vi "air flow calibrator (source setpoint).vi"(4 "State":i16, 5 "Time":dbl format="%.2f", 6 "Sensor Values":dbl[](array[numeric])=[120000.0, 10000.0], 7 "Set Points":dbl[](array[numeric])=[1.0, 22.0, 5e-05]) -> (0 "required data":T1={"Set Point names"=["accumulator volume (L)", "air temperature (C)", "calibration state number", "Source pressure (Pa)"], "required number of setpoints"=4, "required number of sensors"=1, "Sensor names"=["Accumulator pressure (Pa)"]}, 3 "output value":dbl)   [LabVIEW 2019]
uses:
  <vilib>/Analysis/NI_AALPro.lvlib
panel:
  # "Enter the correct information for this control code in the required data structure below. Then make the current value default by right clicking on the border of the data structure."
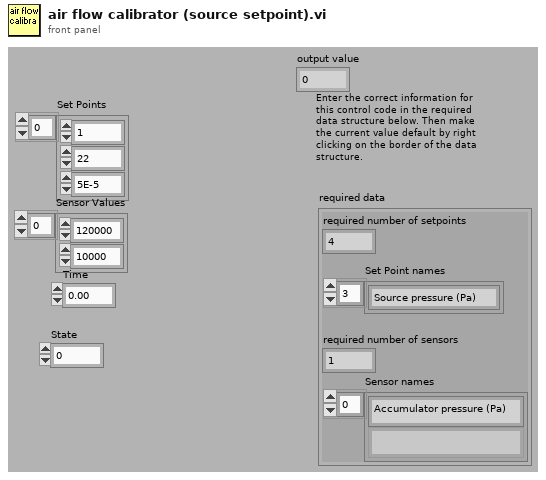
[diagram p1: front panel]
types:
  T1 = cluster{"Set Point names":string[], "required number of setpoints":u8, "required number of sensors":u8, "Sensor names":string[]}
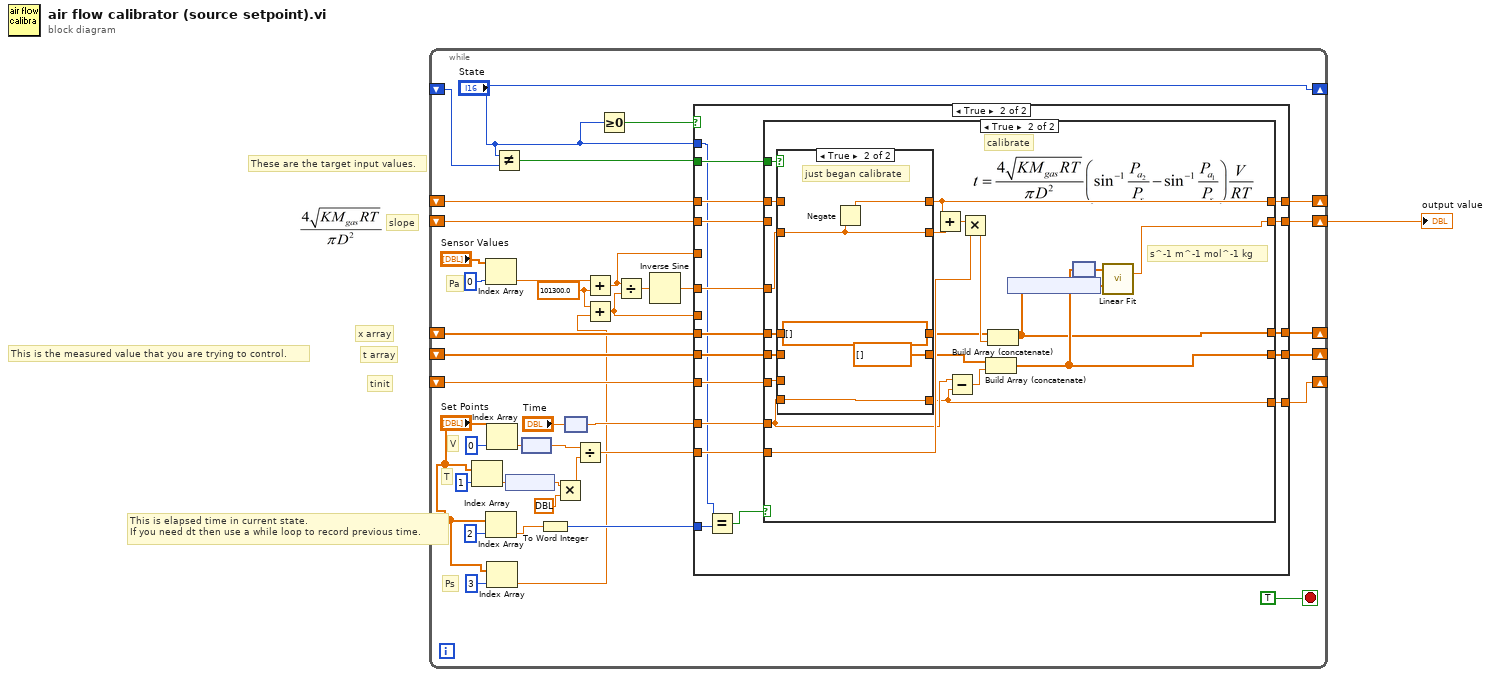
[diagram p0: block diagram]
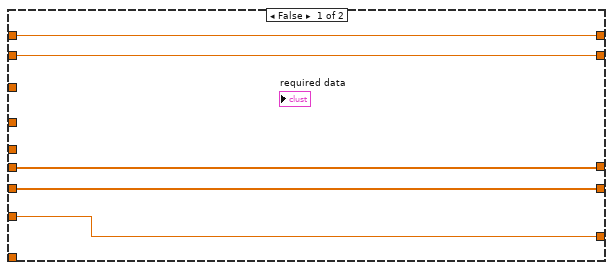
[diagram p2: hidden frame]
diagram:
  # "slope"
  # "tinit"
  # "t array"
  # "x array"
  # "These are the target input values."
  # "This is the measured value that you are trying to control."
  # "This is elapsed time in current state.\nIf you need dt then use a while loop to record previous time."
  n1 = while {
    shift-right: ["State"] -> _
    shift-left: _ -> [w8]
    shift-right: [w39] -> _
    shift-left: _ -> [w38]
    shift-right: [w25] -> _
    shift-left: _ -> [w26]
    shift-right: [w23] -> _
    shift-left: _ -> [w24]
    shift-right: [w21] -> _
    shift-left: _ -> [w20]
    shift-right: [w19] -> w1
    shift-left: _ -> [w18]
    stop <- TRUE stop-if-true
    w12 = 101300.0 ("y")
    # "T"
    # "V"
    # "Ps"
    # "Pa"
    n2 = Index Array(array="Set Points", index=1) -> (element=w33:dbl)
    n3 = Index Array(array="Sensor Values", index=0) -> (element=w15:dbl)
    n4 = Index Array(array="Set Points", index=2) -> (element=w10:dbl)
    n5 = Index Array(array="Set Points", index=0) -> (element=w34:dbl)
    n6 = Index Array(array="Set Points", index=3) -> (element=w3:dbl)
    n7 = Not Equal?(x="State", y=w8) -> (x != y?=w40:bool)
    n8 = node(w33) -> (w31:dbl[unit])
    n9 = node(w34) -> (w32:dbl[unit])
    n10 = To Word Integer(number=w10) -> (16bit integer=w9:i16)
    n11 = Multiply(x=w31, y=ext[unit] 8.3144598000000000003) -> (x*y=w29:ext[unit])
    n12 = node("Time") -> (w22:dbl[unit])
    n13 = Divide(x=w32, y=w29) -> (x/y=w28:ext[unit])
    n14 = Add(x=w15, y=w12) -> (x+y=w13:dbl)
    n15 = Add(x=w12, y=w3) -> (x+y=w14:dbl)
    n16 = Greater Or Equal To 0?(x="State") -> (x >= 0?=w7:bool)
    n17 = Divide(x=w13, y=w14) -> (x/y=w37:dbl)
    n18 = Inverse Sine(1:w37) -> (0:w36:dbl)
    n19 = case shown="True" w7 {
      tunnel: w40 -> [_ w63]
      tunnel: w36 -> [_ w62]
      tunnel: [w45 w60] -> w39
      tunnel: w38 -> [w45 w61]
      tunnel: w28 -> [_ w59]
      tunnel: w22 -> [_ w53]
      tunnel: w26 -> [w44 w58]
      tunnel: [w44 w55] -> w25
      tunnel: w24 -> [w43 w57]
      tunnel: [w43 w56] -> w23
      tunnel: [w42 w52] -> w21
      tunnel: w20 -> [w42 w54]
      tunnel: [w46 w51] -> w19
      tunnel: w18 -> [w46 w48]
      tunnel: w13 -> [_ _]
      tunnel: w14 -> [_ _]
      tunnel: w9 -> [_ w50]
      tunnel: "State" -> [_ w47]
      frame False {
      }
      frame True {
        n20 = Equal?(x=w47, y=w50) -> (x = y?=w49:bool)
        n21 = case shown="True" w49 {
          tunnel: w63 -> [_ w89]
          tunnel: w62 -> [_ w88]
          tunnel: w61 -> [w68 w87]
          tunnel: [w68 w86] -> w60
          tunnel: w59 -> [_ w84]
          tunnel: w58 -> [w66 w80]
          tunnel: w57 -> [w65 w78]
          tunnel: [w65 w77] -> w56
          tunnel: [w66 w76] -> w55
          tunnel: w54 -> [w64 w75]
          tunnel: w53 -> [_ w74]
          tunnel: [w64 w73] -> w52
          tunnel: [w67 w69] -> w51
          tunnel: w48 -> [w67 _]
          frame False {
          }
          frame True {
            # "s^-1 m^-1 mol^-1 kg"
            # "calibrate"
            n22 = case shown="True" w89 {
              tunnel: w88 -> [w93 w98]
              tunnel: [w94 w99] -> w86
              tunnel: w87 -> [w94 _]
              tunnel: [w93 w98] -> w83
              tunnel: [w92 ext[unit][] []] -> w81
              tunnel: w80 -> [w92 _]
              tunnel: [w91 dbl[unit][] []] -> w79
              tunnel: w78 -> [w91 _]
              tunnel: [w90 w95] -> w73
              tunnel: w74 -> [_ w95]
              tunnel: w75 -> [w90 _]
              frame False {
              }
              frame True {
                # "just began calibrate"
                n23 = Negate(x=w98) -> (-x=w99:dbl)
              }
            }
            n24 = Add(x=w86, y=w83) -> (x+y=w85:dbl)
            n25 = Subtract(x=w74, y=w73) -> (x-y=w72:dbl[unit])
            n26 = Multiply(x=w85, y=w84) -> (x*y=w82:ext[unit])
            n27 = Build Array (concatenate)(w79, w72) -> (w77:dbl[unit][])
            n28 = Build Array (concatenate)(w81, w82) -> (w76:ext[unit][])
            n29 = node(w76) -> (w70:ext[])
            n30 = node(w77) -> (w71:dbl[])
            n31 = call <vilib>:"Linear Fit.vi"("Y"=w71, "X"=w70) -> ("slope"=w69:dbl)  [unwired: 9 in, 4 out]
          }
        }
      }
    }
  }
  "output value" <- w1
